vi "Test_Aerotech.vi"() -> ()   [LabVIEW 2009]
uses:
  Controls/AerotechTarget.ctl
panel:
  out "Positions":cluster{dbl, "Position":dbl}(graph)
  in  "Velocity":dbl
  in  "Position":dbl
  out "AEROTECH.ACTUAL":T1
  in  "stop":bool
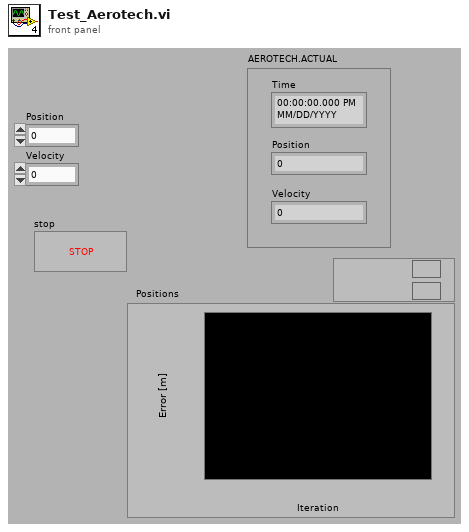
[diagram p1: front panel]
types:
  T1 = typedef "AerotechTarget.ctl" = cluster{"Time":timestamp, "Position":dbl, "Velocity":dbl}
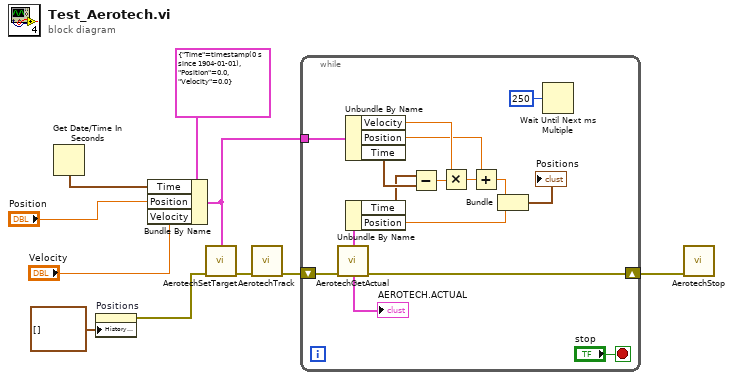
[diagram p0: block diagram]
diagram:
  n1 = Get Date/Time In Seconds() -> (seconds since 1Jan1904=w6:timestamp)
  n2 = property on="Positions" class="WFChart (strict)"("History Data"=cluster{dbl, "Position":dbl}[] []) -> (error out=w1:errorcluster)  [unwired: 2 in, 1 out]
  n3 = Bundle By Name(cluster=T1 {"Time"=timestamp(0 s since 1904-01-01), "Position"=0.0, "Velocity"=0.0} ("AEROTECH.TARGET"), "Time"=w6, "Position"="Position", "Velocity"="Velocity") -> (w3:T1)
  n4 = call "AerotechSetTarget.vi"("error in (no error)"=w1, "AEROTECH.TARGET"=w3) -> ("error out"=w10:errorcluster)  [unwired: 3 in]
  n5 = call "AerotechTrack.vi"("error in (no error)"=w10) -> ("error out"=w9:errorcluster)  [unwired: 10 in]
  n6 = while {
    shift-right: [w23] -> w8
    shift-left: w9 -> [w25]
    tunnel: w3 -> [w22]
    stop <- "stop" stop-if-true
    n7 = call "AerotechGetActual.vi"("error in (no error)"=w25) -> ("error out"=w23:errorcluster, "AEROTECH.ACTUAL"=w21:T1)  [unwired: 3 in]
    "AEROTECH.ACTUAL" <- w21
    n8 = Unbundle By Name(w22) -> ("Velocity"=w18:dbl, "Position"=w15:dbl, "Time"=w20:timestamp)
    n9 = Unbundle By Name(w21) -> ("Time"=w19:timestamp, "Position"=w12:dbl)
    n10 = Subtract(x=w19, y=w20) -> (x-y=w17:dbl)
    n11 = Multiply(x=w18, y=w17) -> (x*y=w16:dbl)
    n12 = Add(x=w15, y=w16) -> (x+y=w13:dbl)
    n13 = Bundle(w13, "Position"=w12) -> (→"Positions":cluster{dbl, "Position":dbl})  [unwired: 1 in]
    n14 = Wait Until Next ms Multiple(millisecond multiple=u32 250) -> ()  [unwired: 1 out]
  }
  n15 = call "AerotechStop.vi"("error in (no error)"=w8) -> ()  [unwired: 10 in, 1 out]
